vi "Forward_Kinematics (geo and matrix).vi"(7 "q2":dbl(slide)=65.928599536276 scale=0.0..200.0, 8 "q1":dbl(slide)=-18.502559699737844 scale=0.0..200.0, 9 "geometry?":bool=TRUE, 10 "arms":T2(array[cluster])=[{"Translation"={"X"=0.0, "Y"=0.0, "Z"=0.0}, "Axis"=enum."z", "Angle (degrees)"=20.0}, {"Translation"={"X"=30.0, "Y"=0.0, "Z"=0.0}, "Axis"=enum."z", "Angle (degrees)"=-40.0}, {"Translation"={"X"=35.0, "Y"=0.0, "Z"=0.0}, "Axis"=enum."z", "Angle (degrees)"=0.0}] {"Angle (degrees)" scale=0.0..180.0}, 11 "new picture":picture) -> (0 "end (2D)":cluster{"x":dbl, "y":dbl}={"x"=161.99999999999997, "y"=64.00000000000003}, 1 "end effector":cluster{"X":dbl, "Y":dbl}={"X"=38.00000000000003, "Y"=135.99999999999997}, 3 "2D Picture":picture)   [LabVIEW 2024]
uses:
  <vilib>/Analysis/Matrix/Datatypes/RealMatrix.ctl
  <vilib>/Analysis/baseanly.llb/Real A x B.vi
  <vilib>/Analysis/NI_AALBase.lvlib
  <vilib>/Analysis/Matrix/NI_Matrix.lvlib
panel:
  out "output variable 2":dbl=135.99999999999997
  out "output variable":dbl=38.00000000000003
  out "Array":T1(array[cluster])=[{"Real Matrix Element"=0.0, "Real Matrix Element"=0.0}, {"Real Matrix Element"=28.190778623577252, "Real Matrix Element"=10.260604299770062}, {"Real Matrix Element"=61.080020351084045, "Real Matrix Element"=-1.710100716628343}]
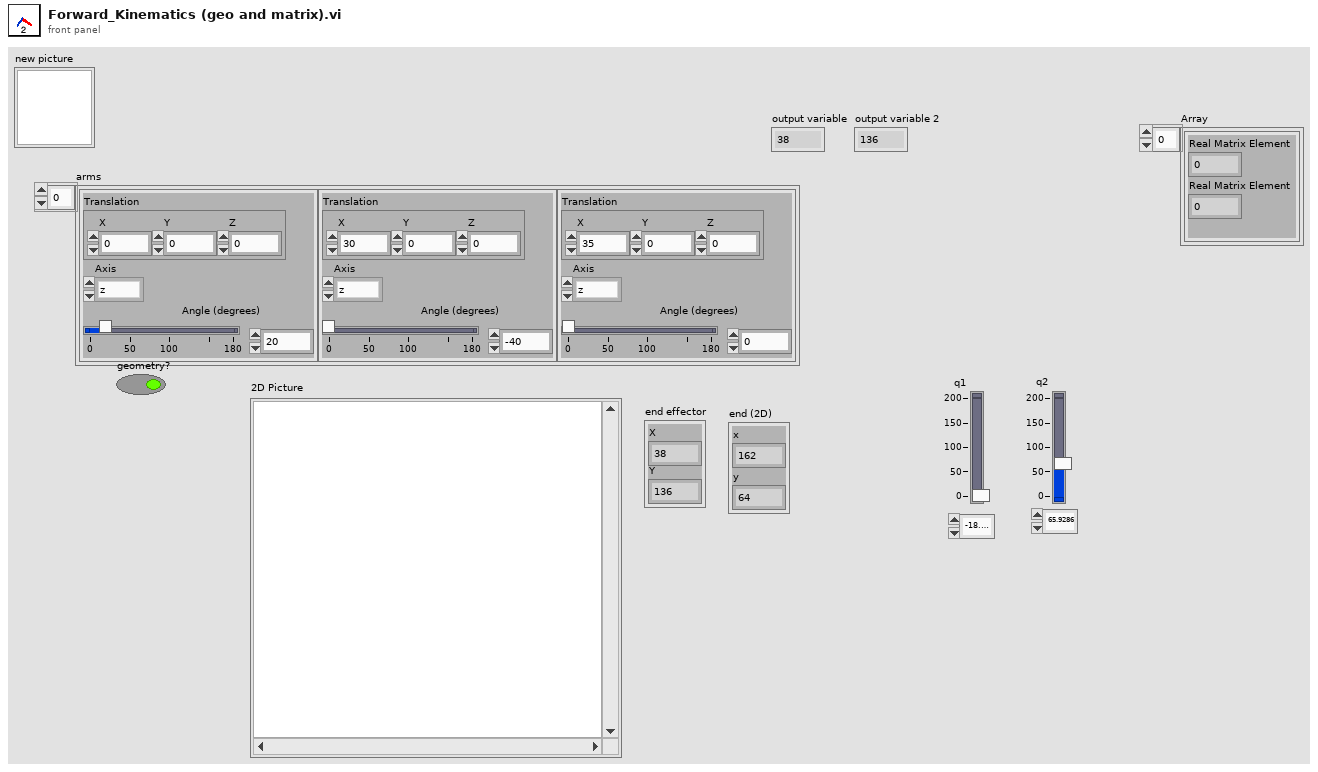
[diagram p1: front panel]
types:
  T1 = cluster{"Real Matrix Element":dbl, "Real Matrix Element":dbl}[]
  T2 = cluster{"Translation":cluster{"X":dbl, "Y":dbl, "Z":dbl}, "Axis":enum16{"x", "y", "z"}, "Angle (degrees)":dbl}[]
  T3 = typedef "NI_Matrix.lvlib/RealMatrix.ctl" = dbl[][]
  T4 = cluster{"Real Matrix Element":dbl, "Real Matrix Element":dbl}
  T5 = cluster{"Width":u16, "Style":enum32{"Solid", "Dash", "Dot", "DashDot", "DashDotDot"}}
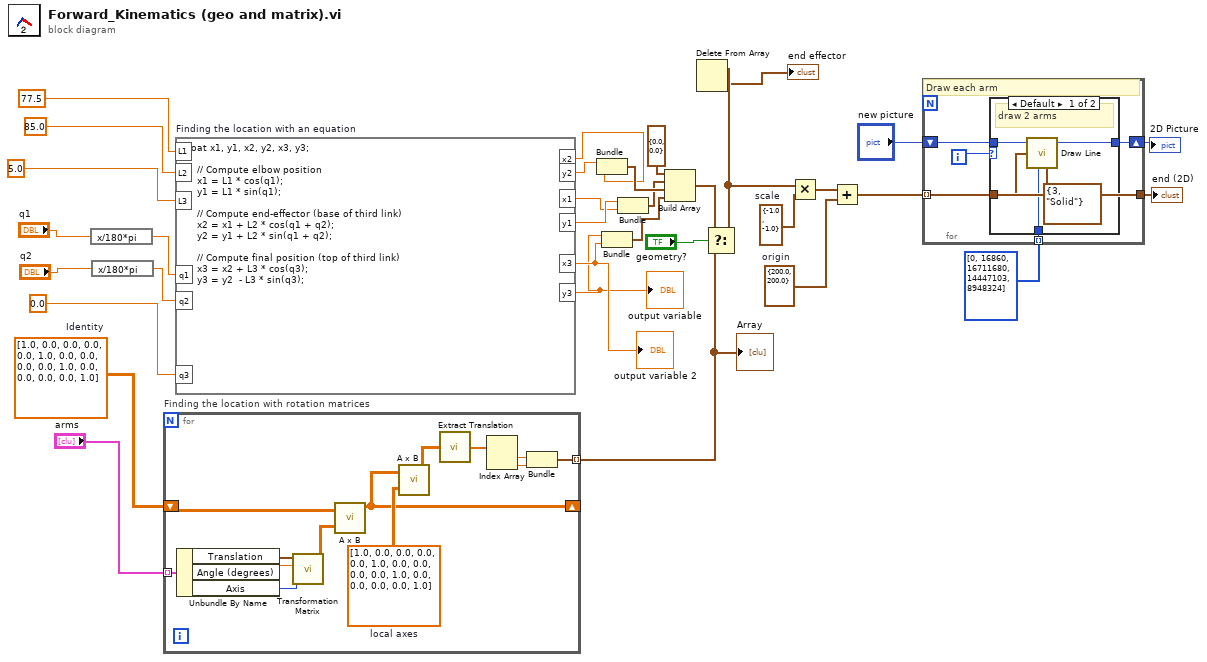
[diagram p0: block diagram]
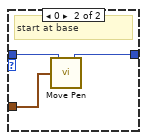
[diagram p2: hidden frame]
diagram:
  w25 = T3 [[1.0, 0.0, 0.0, 0.0], [0.0, 1.0, 0.0, 0.0], [0.0, 0.0, 1.0, 0.0], [0.0, 0.0, 0.0, 1.0]]  # Identity
  w30 = cluster{"x":dbl, "y":dbl} {"x"=-1.0, "y"=-1.0}  # scale
  w29 = cluster{"x":dbl, "y":dbl} {"x"=200.0, "y"=200.0}  # origin
  n1 = expression code="x/180*pi"("q1") -> (w15:dbl)
  n2 = expression code="x/180*pi"("q2") -> (w16:dbl)
  n3 = for "Finding the location with rotation matrices" {
    tunnel: "arms" -> [w41] mode=indexing
    shift-right: [w39] -> _
    shift-left: w25 -> [w40]
    tunnel: [w34] -> w24 mode=indexing
    w42 = T3 [[1.0, 0.0, 0.0, 0.0], [0.0, 1.0, 0.0, 0.0], [0.0, 0.0, 1.0, 0.0], [0.0, 0.0, 0.0, 1.0]]  # local axes
    n4 = Unbundle By Name(w41) -> ("Translation"=w46:cluster{"X":dbl, "Y":dbl, "Z":dbl}, "Angle (degrees)"=w45:dbl, "Axis"=w44:enum16{"x", "y", "z"})
    n5 = call <userlib>:"Transformation Matrix.vi"("Axis"=w44, "Angle (degrees)"=w45, "Translation"=w46) -> ("Transformation Matrix"=w43:T3)  [unwired: 8 in]
    n6 = call-poly <vilib>:"A x B.vi"("B"=w43, "A"=w40) -> ("A x B"=w39:T3)  [unwired: 1 out]
    n7 = call-poly <vilib>:"A x B.vi"("B"=w42, "A"=w39) -> ("A x B"=w38:T3)  [unwired: 1 out]
    n8 = call <userlib>:"Extract Translation.vi"("Transformation matrix"=w38) -> ("translation"=w37:dbl[])
    n9 = Index Array(array=w37) -> (element #1=w36:dbl, element #2=w35:dbl)  [unwired: 2 in]
    n10 = Bundle("Real Matrix Element"=w36, "Real Matrix Element"=w35) -> (w34:T4)  [unwired: 1 in]
  }
  "Array" <- w24
  n11 = formula code="float x1, y1, x2, y2, x3, y3;\n\n    // Compute elbow position\n    x1 = L1 * cos(q1);\n    y1 = L1 * sin(q1);\n\n    // Compute end-effector (base of third link)\n    x2 = x1 + L2 * cos(q1 + q2);\n    y2 = y1 + L2 * sin(q1 + q2);\n\n    // Compute final position (top of third link)\n    x3 = x2 + L3 * cos(q3);\n    y3 = y2  - L3 * sin(q3);" "Finding the location with an equation"("q1"=w15, "L1"=77.5 ("q3"), "L2"=85.0 ("q3"), "q2"=w16, "q3"=0.0, "L3"=5.0 ("q3")) -> ("x1"=w3:dbl, "y1"=w4:dbl, "x2"=w5:dbl, "y2"=w6:dbl, "x3"=w2:dbl, "y3"=w1:dbl)
  "output variable" <- w1
  "output variable 2" <- w2
  n12 = Bundle(w6, w5) -> (w9:cluster{dbl, dbl})  [unwired: 1 in]
  n13 = Bundle(w1, w2) -> (w10:cluster{dbl, dbl})  [unwired: 1 in]
  n14 = Bundle(w4, w3) -> (w8:cluster{dbl, dbl})  [unwired: 1 in]
  n15 = Build Array(cluster{"x":dbl, "y":dbl} {"x"=0.0, "y"=0.0} ("y"), w8, w9, w10) -> (w23:cluster{"x":dbl, "y":dbl}[])
  n16 = Select(t=w23, s="geometry?", f=w24) -> (s? t:f=w21:T1)
  n17 = Delete From Array(array=w21) -> (deleted portion=→"end effector":T4)  [unwired: 2 in, 1 out]
  n18 = Multiply(x=w21, y=w30) -> (x*y=w28:cluster{dbl, dbl}[])
  n19 = Add(x=w28, y=w29) -> (x+y=w27:cluster{dbl, dbl}[])
  n20 = for {
    shift-right: [w49] -> w32
    shift-left: "new picture" -> [w50]
    tunnel: u32[] [0, 16860, 16711680, 14447103, 8948324] -> [w48] mode=indexing
    tunnel: w27 -> [w47] mode=indexing
    tunnel: [w47] -> w19
    i -> [w51]
    # "Draw each arm"
    n21 = case shown="Default" w51 {
      tunnel: w50 -> [w56 w59]
      tunnel: [w55 w58] -> w49
      tunnel: w47 -> [w54 w57]
      tunnel: w48 -> [w53 _]
      frame Default {
        # "draw 2 arms"
        n22 = call <vilib>:"Draw Line.vi"("picture"=w56, "end point"=w54, "color(black)"=w53, "pen"=T5 {"Width"=3, "Style"=enum."Solid"}) -> ("new picture"=w55:picture)  [unwired: 5 in]
      }
      frame 0 {
        # "start at base"
        n23 = call <vilib>:"Move Pen.vi"("new position"=w57, "picture"=w59) -> ("new picture"=w58:picture)  [unwired: 3 in]
      }
    }
  }
  "2D Picture" <- w32
  "end (2D)" <- w19
